vi "example.vi"() -> ()   [LabVIEW 2019]
uses:
  <vilib>/DAQmx/read.llb/DAQmx Read (Analog 1D Wfm NChan NSamp).vi
  <vilib>/DAQmx/create/channels.llb/DAQmx Create Channel (AI-Voltage-Basic).vi
  <vilib>/DAQmx/configure/timing.llb/DAQmx Timing (Sample Clock).vi
  <vilib>/DAQmx/configure/trigger.llb/DAQmx Start Trigger (Analog Edge).vi
  <vilib>/DAQmx/configure/task.llb/DAQmx Configure Logging (TDMS).vi
  <vilib>/DAQmx/miscellaneous.llb/DAQmx Fill In Error Info.vi
  <resource>/objmgr/daqmx.rc
panel:
  out "Waveform Graph":waveform(dbl)[](graph)=[{"t0"=timestamp(3656727970.737722 s since 1904-01-01), "dt"=4.999999999999959e-06, "Y"=array[4000 elements], "attributes"=variant("NI_ChannelName"=variant(string "NI_9775/ai0"), "NI_UnitDescription"=variant(string "Volts"))}, {"t0"=timestamp(3656727970.737722 s since 1904-01-01), "dt"=4.999999999999959e-06, "Y"=array[4000 elements], "attributes"=variant("NI_ChannelName"=variant(string "NI_9775/ai1"), "NI_UnitDescription"=variant(string "Volts"))}]
  in  "TDMS File":path=path "D:/Python/nitdms/tests/tdms_files/example.tdms"
  out "Error Out":errorcluster
  in  "NI-9435":tag="NI_9435/port0/line0:3"
  in  "NI-9775":tag="NI_9775/ai0:1"
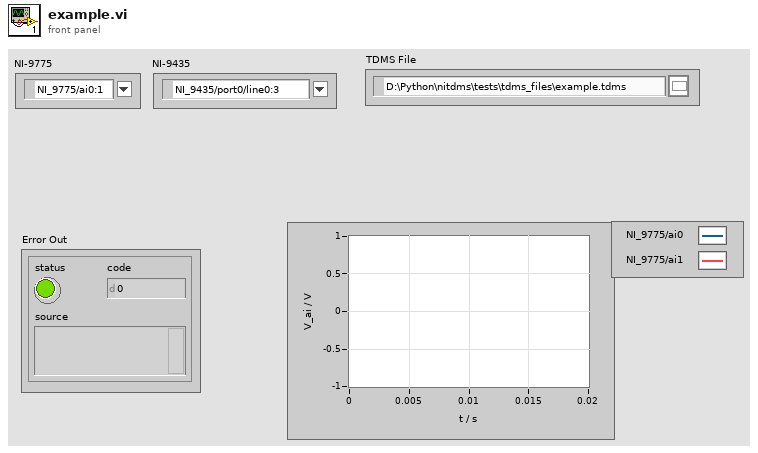
[diagram p1: front panel]
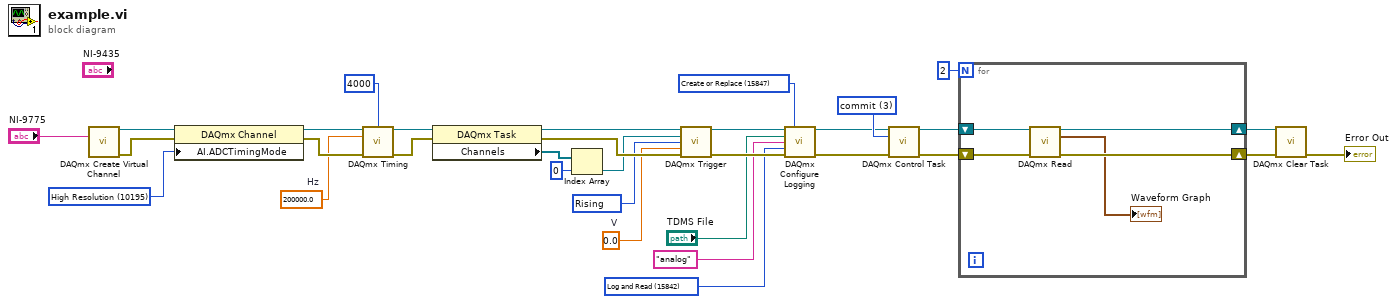
[diagram p0: block diagram]
diagram:
  w6 = 15842 items=["Off"=10231, "Log"=15844, "Log and Read"=15842] ("logging mode")
  w9 = 15847 items=["Open"=10437, "Open or Create"=15846, "Create or Replace"=15847, "Create"=15848] ("operation")
  w18 = 3 items=["verify"=2, "reserve"=4, "commit"=3, "unreserve"=5, "abort"=6] ("action")
  w19 = 0.0  # V
  w20 = 10280 items=["Rising"=10280, "Falling"=10171] ("slope")
  w26 = 200000.0  # Hz
  w29 = 10195 items=["Automatic"=16097, "High Resolution"=10195, "High Speed"=14712, "Best 50 Hz Rejection"=14713, "Best 60 Hz Rejection"=14714, "Custom"=10137] ("AI.ADCTimingMode")
  n1 = call-poly <vilib>:"DAQmx Create Virtual Channel.vi"("physical channels"="NI-9775") -> ("task out"=w31:refnum<k21>, "error out"=w30:errorcluster)  [unwired: 13 in]
  n2 = property class="DAQmx Channel"(reference=w31, error in=w30, "AI.ADCTimingMode"=w29) -> (reference out=w28:refnum<k21>, error out=w27:errorcluster)
  n3 = call-poly <vilib>:"DAQmx Timing.vi"("task/channels in"=w28, "samples per channel"=4000, "rate"=w26, "error in"=w27) -> ("task out"=w15:refnum<k21>, "error out"=w16:errorcluster)  [unwired: 10 in]
  n4 = property class="DAQmx Task"(reference=w15, error in=w16) -> (reference out=w22:refnum<k21>, error out=w23:errorcluster, "Channels"=w25:refnum<k21>[])
  n5 = Index Array(array=w25, index=0) -> (element=w21:refnum<k21>)
  n6 = call-poly <vilib>:"DAQmx Trigger.vi"("task/channels in"=w22, "source"=w21, "slope"=w20, "level"=w19, "error in"=w23) -> ("task out"=w10:refnum<k21>, "error out"=w11:errorcluster)  [unwired: 9 in]
  n7 = call-poly <vilib>:"DAQmx Configure Logging.vi"("task/channels in"=w10, "operation"=w9, "file path"="TDMS File", "group name"="analog", "logging mode"=w6, "error in"=w11) -> ("task out"=w4:refnum<k21>, "error out"=w5:errorcluster)  [unwired: 8 in]
  n8 = call <vilib>:"DAQmx Control Task.vi"("task/channels in"=w4, "action"=w18, "error in"=w5) -> ("task out"=w2:refnum<k21>, "error out"=w3:errorcluster)  [unwired: 11 in]
  n9 = for {
    N: 2 -> [_]
    shift-right: [w37] -> w14
    shift-left: w3 -> [w34]
    shift-right: [w36] -> w13
    shift-left: w2 -> [w33]
    n10 = call-poly <vilib>:"DAQmx Read.vi"("task/channels in"=w33, "error in"=w34) -> ("task out"=w36:refnum<k21>, "data"=→"Waveform Graph":waveform(dbl)[], "error out"=w37:errorcluster)  [unwired: 11 in]
  }
  n11 = call <vilib>:"DAQmx Clear Task.vi"("task in"=w13, "error in"=w14) -> ("error out"=→"Error Out":errorcluster)  [unwired: 13 in]
